vi "Velocity Low Check.vi"(7 "Initialize":bool, 11 "Shoulder Velocity":i32) -> (3 "Velocity Low for Time":bool)   [LabVIEW 2018]
uses:
  <vilib>/ptbypt/NI_PtbyPt.lvlib
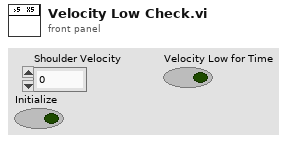
[diagram p1: front panel]
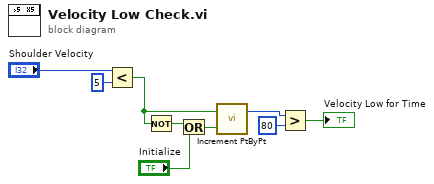
[diagram p0: block diagram]
diagram:
  n1 = Less?(x="Shoulder Velocity", y=5) -> (x < y?=w7:bool)
  n2 = Not(x=w7) -> (.not. x?=w3:bool)
  n3 = Or(x=w3, y="Initialize") -> (x .or. y?=w2:bool)
  n4 = call <vilib>:"Increment PtByPt.vi"("initialize"=w2, "activate"=w7) -> ("counter"=w5:u32)  [unwired: 1 out]
  n5 = Greater?(x=w5, y=80) -> (0:→"Velocity Low for Time":bool)
